vi "patientUpdateView.vi"() -> ()   [LabVIEW 2019]
doc: "40"
uses:
  03_Home/controller/logoutBtn.ctl
  03_Home/controller/exitBtn.ctl
  03_Home/controller/pannelState.ctl
  <vilib>/Utility/miscctls.llb/LVPointTypeDef.ctl
  subVI/patients_state.ctl
  globalValue.vi
panel:
  in  "patients_weight":dbl format="%.1f"
  in  "patients_age":dbl
  in  "patients_height":dbl format="%.1f"
  in  "patients_birthdate":dbl format="%<%Y-%m-%d>T"
  in  "cancelBtn":bool
  in  "patients_gender":string(combo)
  in  "backPage":bool
  in  "patients_info":string
  in  "patients_address":string
  in  "patients_phone":string
  in  "patients_email":string
  in  "patients_nm":string
  in  "updateBtn":bool
  in  "deleteBtn":bool
  out "patients_id":string
  out "userDetailInfo":string[](array[string])
  in  "Help Button":bool
  in  "LogOut Button":T1
  in  "Exit Button":T2
  out "userNm":string
  # "|"
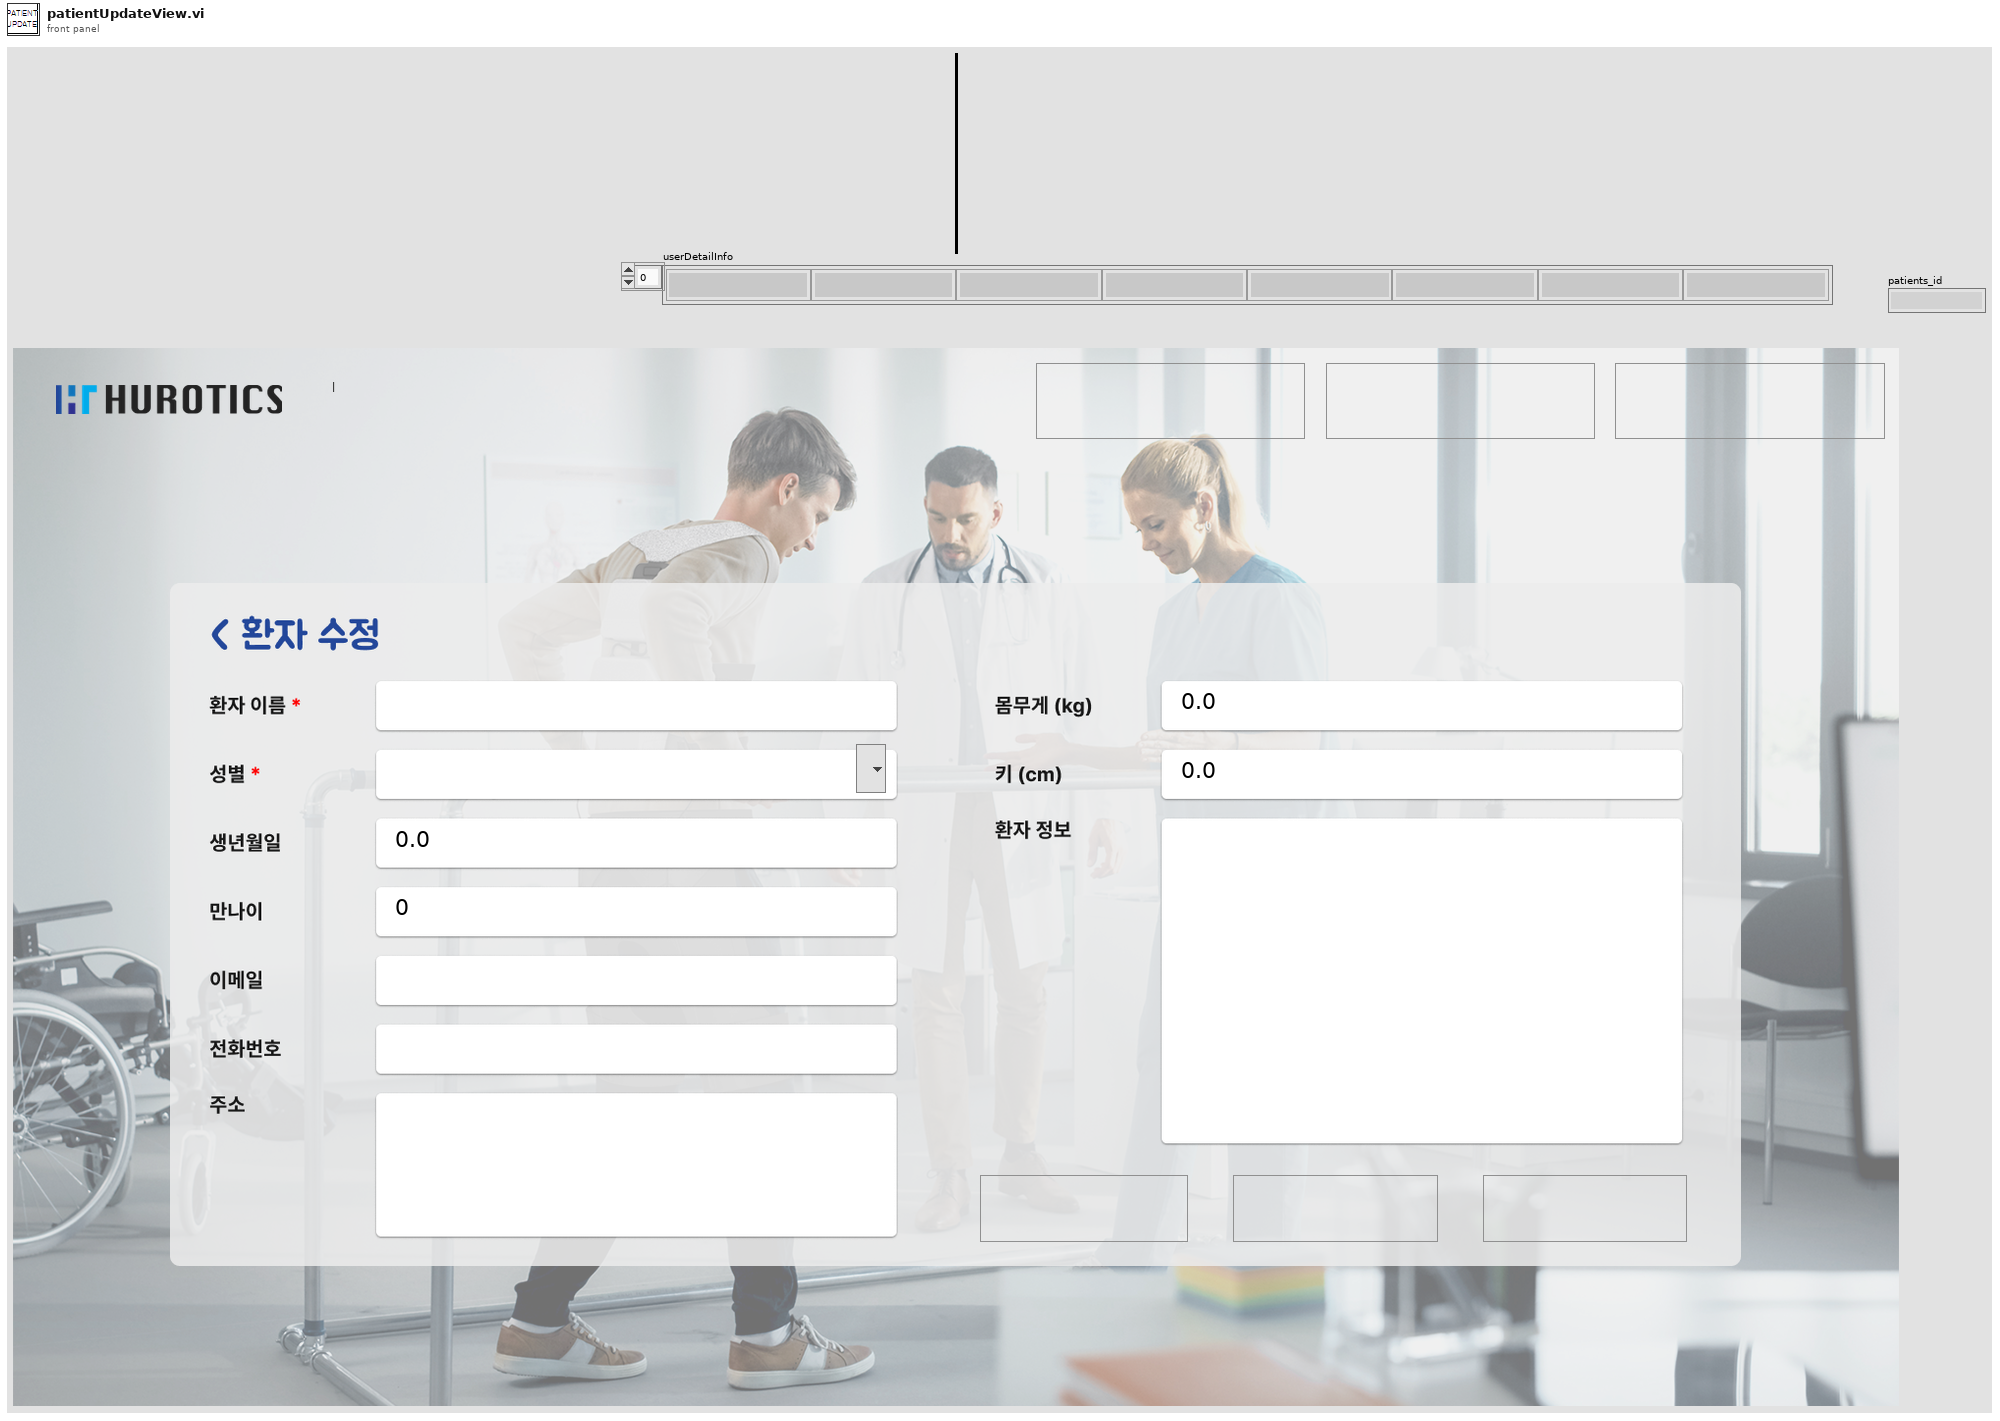
[diagram p1: front panel]
types:
  T1 = typedef "logoutBtn.ctl" = bool
  T2 = typedef "exitBtn.ctl" = bool
  T3 = typedef "pannelState.ctl" = enum16{"Init", "LogIn", "SignUpView", "Home", "Management_patientList", "Management_patientTrashtList", "Management_patientCreate", "Management_patientUpdate", "Management_patientTraining", "Management_patientTrainingDetail", "H-MEDI PatientList", "H-MEDI HardwareCtl", "Adjust", "FineTuning", "UserList", "UserDetail", "Exit"}
  T4 = typedef "LVPointTypeDef.ctl" = cluster{"Horizontal":i16, "Vertical":i16}
  T5 = enum16{"connection", "create", "getReadList", "getRead", "getCount", "update", "delete", "close"}
  T6 = typedef "patients_state.ctl" = enum16{"connection", "create", "getReadList", "getRead", "getCount", "update", "delete", "trash", "restore", "close"}
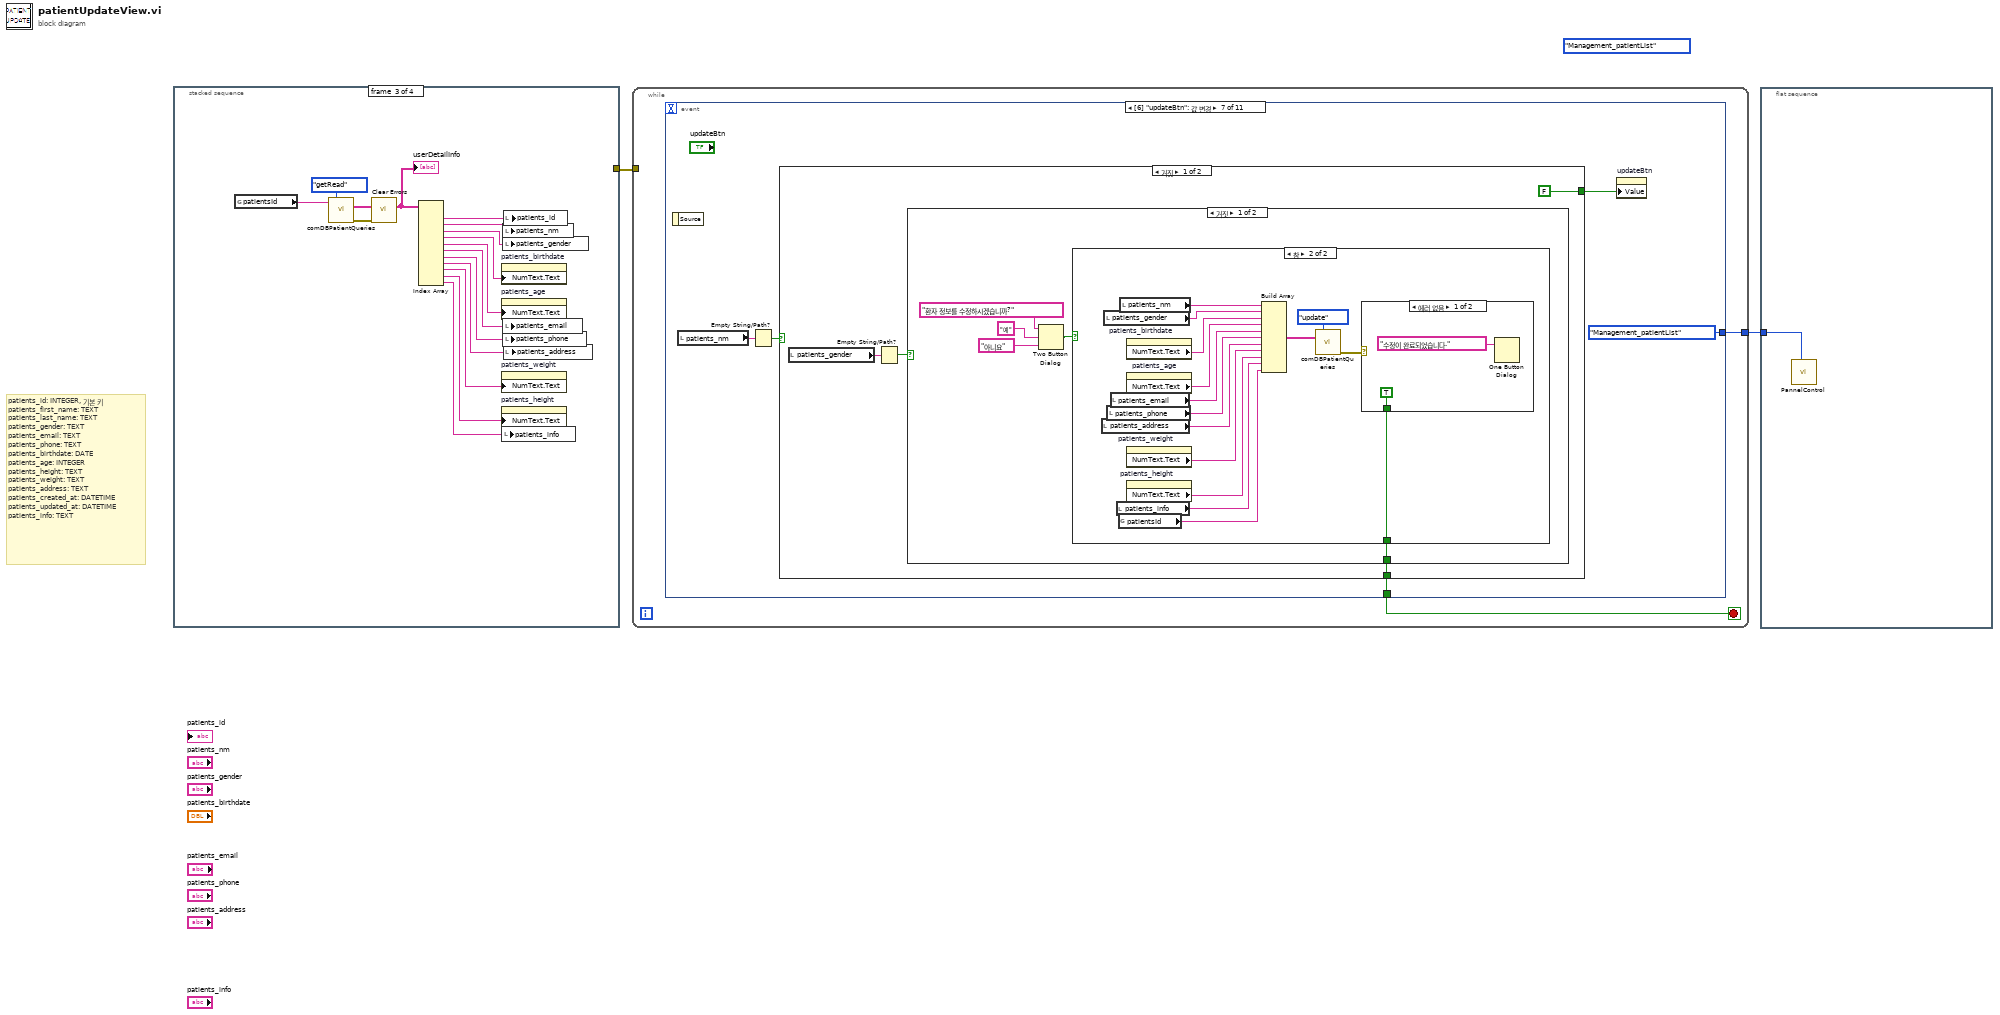
[diagram p0: block diagram]
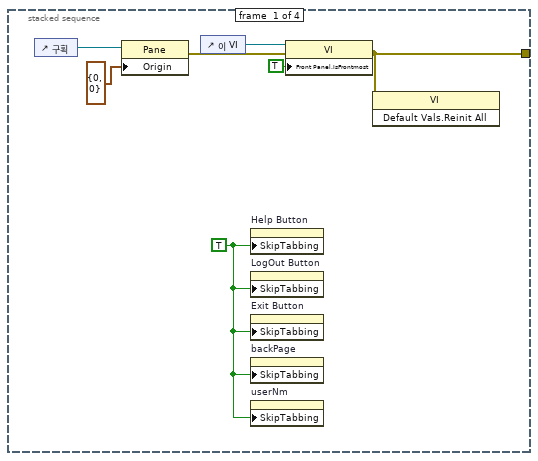
[diagram p2: hidden frame]
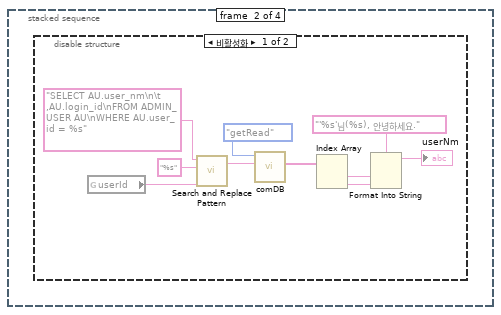
[diagram p3: hidden frame]
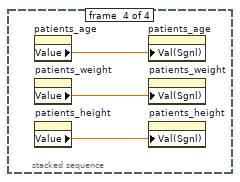
[diagram p5: hidden frame]
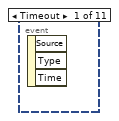
[diagram p6: hidden frame]
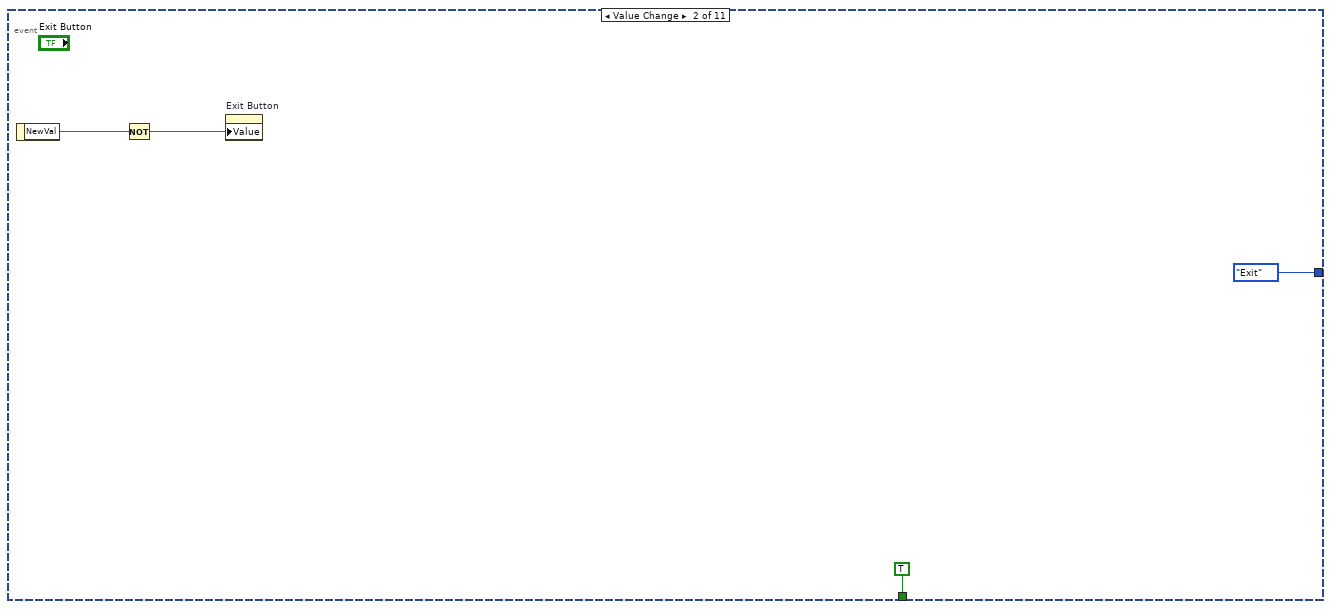
[diagram p7: hidden frame]
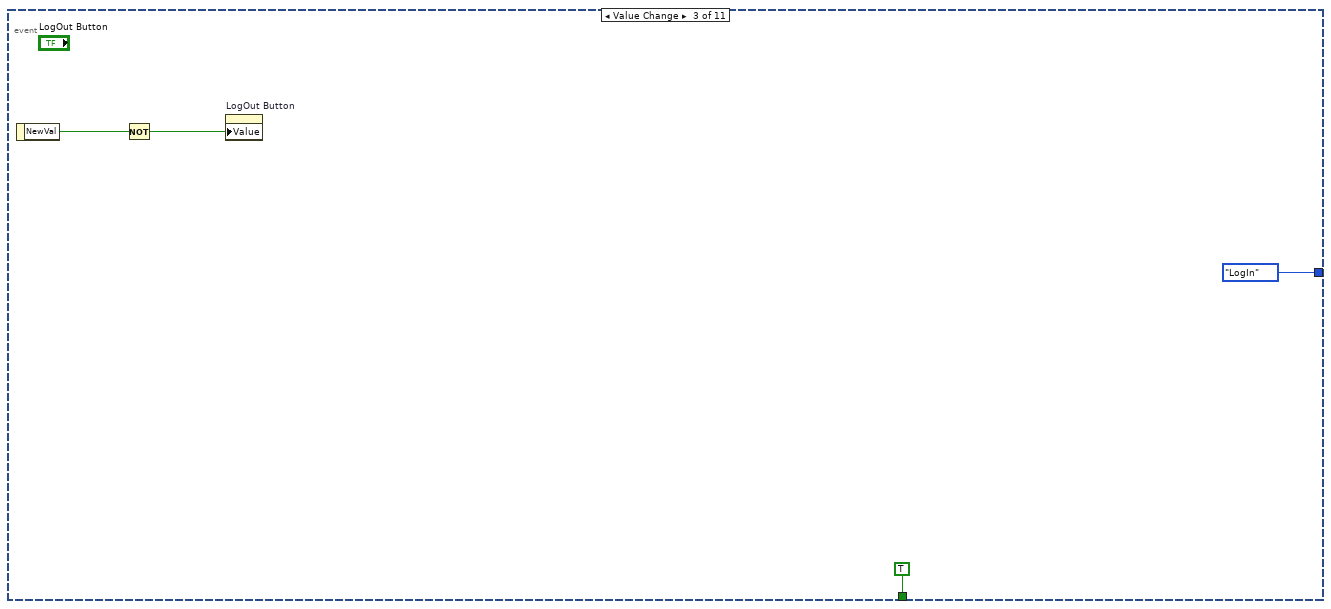
[diagram p8: hidden frame]
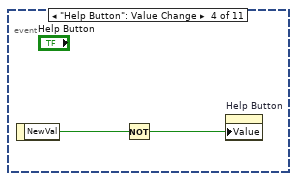
[diagram p9: hidden frame]
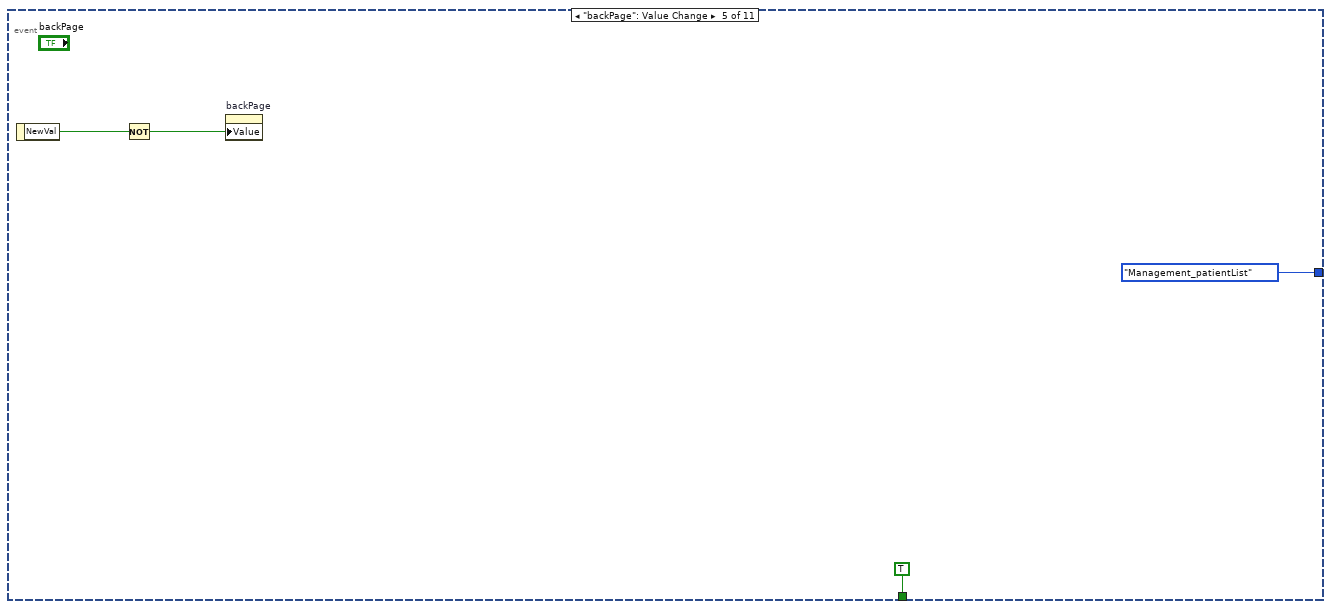
[diagram p10: hidden frame]
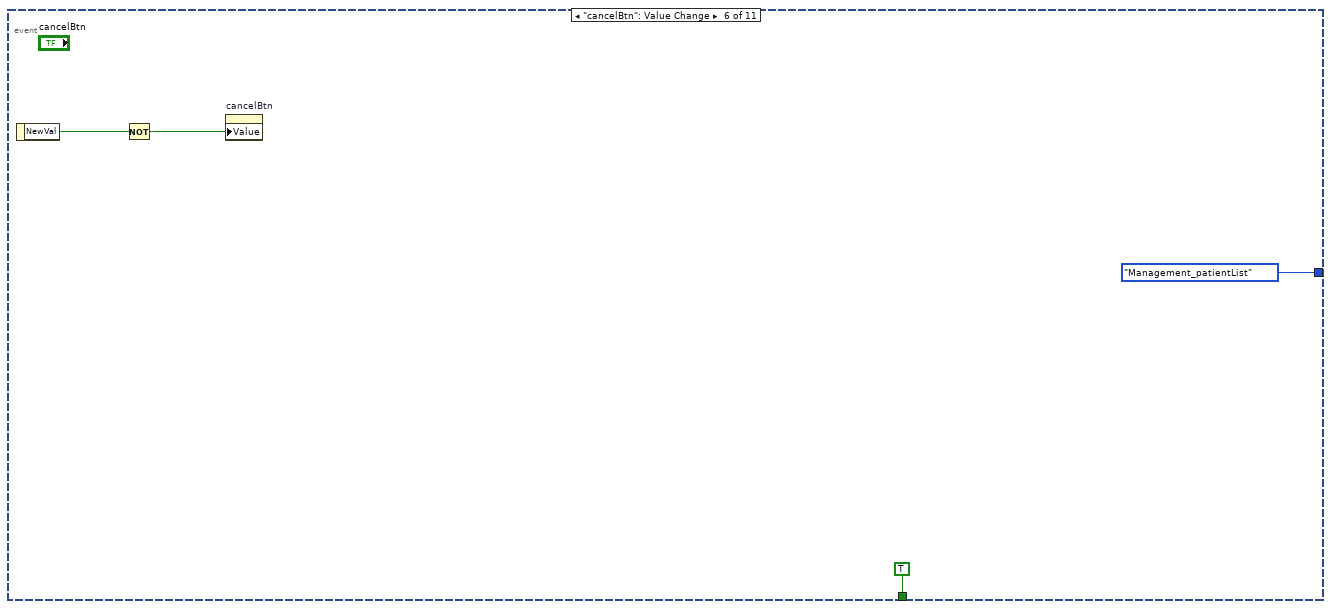
[diagram p11: hidden frame]
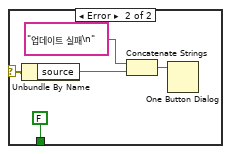
[diagram p13: hidden frame]
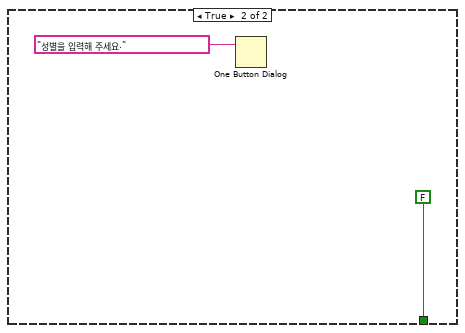
[diagram p14: hidden frame]
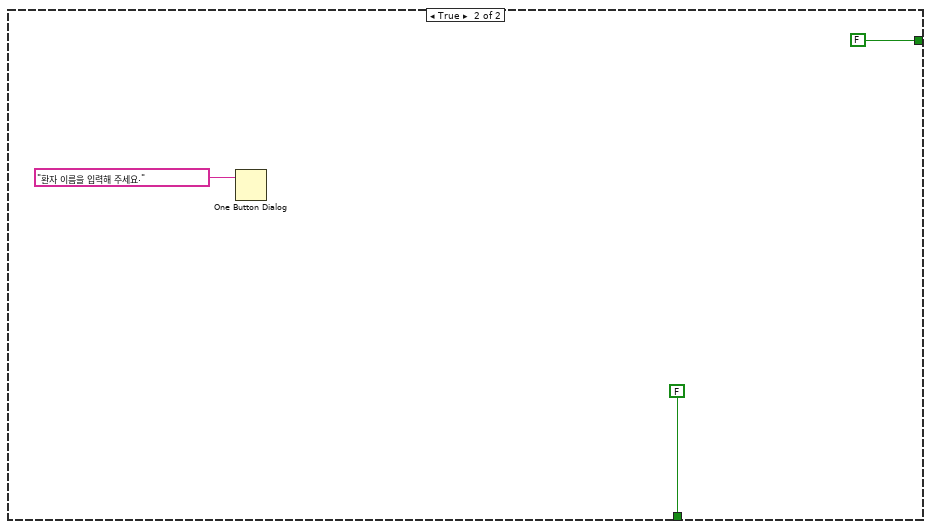
[diagram p15: hidden frame]
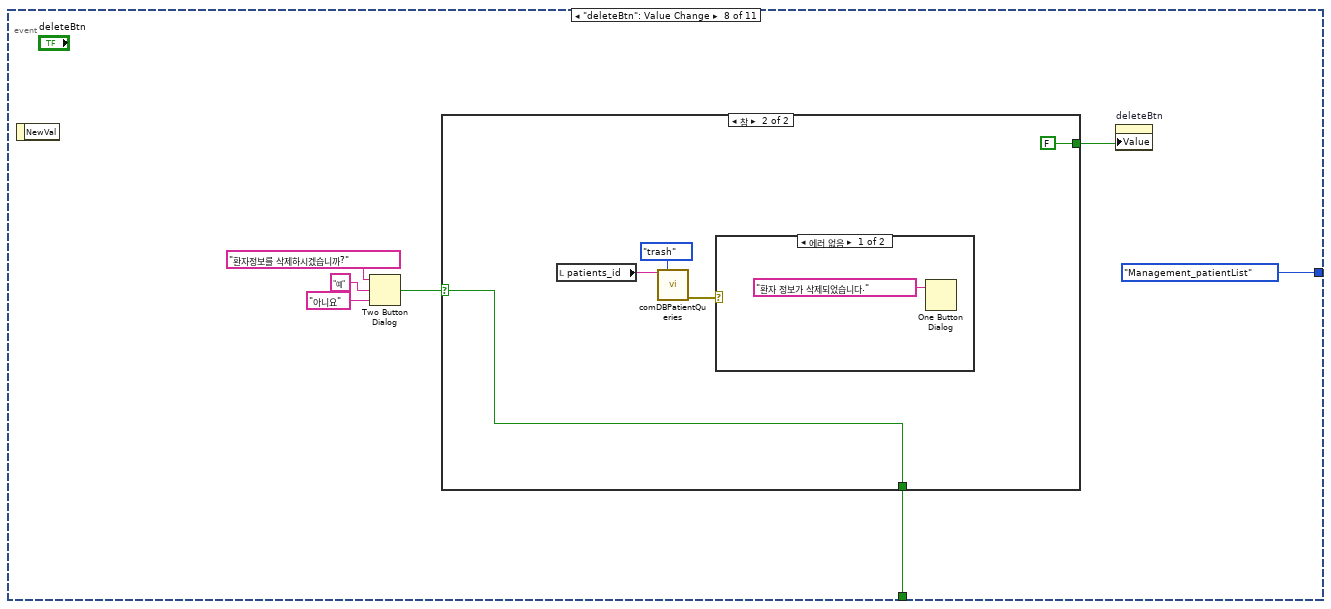
[diagram p16: hidden frame]
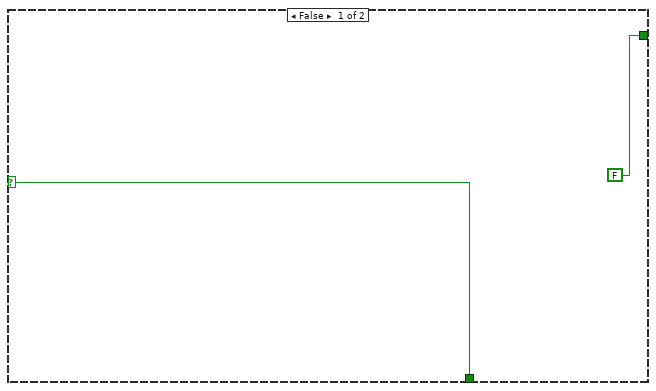
[diagram p17: hidden frame]
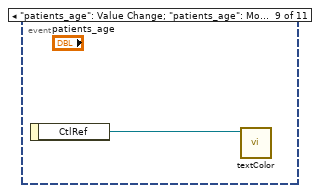
[diagram p19: hidden frame]
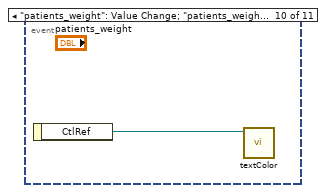
[diagram p20: hidden frame]
diagram:
  (unwired) pannelState."Management_patientList" ("State")
  # "patients_id: INTEGER, 기본 키\npatients_first_name: TEXT\npatients_last_name: TEXT\npatients_gender: TEXT\npatients_email: TEXT\npatients_phone: TEXT\npatients_birthdate: DATE\npatients_age: INTEGER\npatients_height: TEXT\npatients_weight: TEXT\npatients_address: TEXT\npatients_created_at: DATETIME\npatients_updated_at: DATETIME\npatients_info: TEXT"
  n1 = stacked-sequence {
    tunnel: [w4 _ _ _] -> w1
    frame #0 {
      w3 = TRUE ("탭으로 이동 시 건너뛰기")
      n2 = control-ref of="구획"() -> (w7:refnum<vi>)
      n3 = property class="Pane"(reference=w7, "Origin"=T4 {"Horizontal"=0, "Vertical"=0} ("원점")) -> (error out=w5:errorcluster)  [unwired: 1 in, 1 out]
      n4 = control-ref of="이 VI"() -> (w9:refnum<vi>)
      n5 = property on="Help Button" class="Bool (엄격한)"("SkipTabbing"=w3) -> ()  [unwired: 2 in, 2 out]
      n6 = property on="LogOut Button" class="Bool (엄격한)"("SkipTabbing"=w3) -> ()  [unwired: 2 in, 2 out]
      n7 = property on="Exit Button" class="Bool (엄격한)"("SkipTabbing"=w3) -> ()  [unwired: 2 in, 2 out]
      n8 = property on="backPage" class="Bool (엄격한)"("SkipTabbing"=w3) -> ()  [unwired: 2 in, 2 out]
      n9 = property on="userNm" class="Str"("SkipTabbing"=w3) -> ()  [unwired: 2 in, 2 out]
      n10 = property class="VI"(reference=w9, error in=w5, "Front Panel.IsFrontmost"=TRUE ("프런트패널 윈도우:맨 앞으로")) -> (error out=w4:errorcluster)  [unwired: 1 out]
      n11 = invoke class="VI" method="Default Vals.Reinit All"(error in=w4) -> ()  [unwired: 2 in, 3 out]
    }
    frame #1 {
      n12 = disable-structure shown="비활성화" {
        frame Disabled {
          n13 = global read "globalValue.vi" "userId"() -> (w10:string)
          n14 = call <vilib>:"Search and Replace Pattern.vi"("string"="SELECT AU.user_nm\n\t         ,AU.login_id\nFROM ADMIN_USER AU\nWHERE AU.user_id = %s" ("Query"), "regular expression (\"\")"="%s" ("regular expression (\"\")"), "replace string (\"\")"=w10) -> ("result string"=w11:string)  [unwired: 2 in, 1 out]
          n15 = call "comDB.vi"("Query"=w11, "State"=T5."getRead") -> ("result1DArray"=w17:string[])  [unwired: 5 in, 3 out]
          n16 = Index Array(array=w17) -> (element #1=w16:string, element #2=w15:string)  [unwired: 2 in]
          n17 = Format Into String(format string="'%s'님(%s), 안녕하세요." ("문자열"), w16, w15) -> (resulting string=→"userNm":string)  [unwired: 2 in, 1 out]
        }
        frame Enabled {
        }
      }
    }
    frame #2 {
      n18 = global read "globalValue.vi" "patientsId"() -> (w20:string)
      n19 = call "comDBPatientQueries.vi"("id"=w20, "State"=patients_state."getRead") -> ("result1DArray"=w28:string[], "error out"=w27:errorcluster)  [unwired: 10 in, 2 out]
      "userDetailInfo" <- w28
      n20 = call <vilib>:"Clear Errors.vi"("error in (no error)"=w27) -> ()  [unwired: 5 in, 2 out]
      n21 = Index Array(array=w28) -> (element #1=w29:string, element #2=w34:string, element #3=w26:string, element #4=w24:string, element #5=w23:string, element #6=w33:string, element #7=w32:string, element #8=w31:string, element #9=w22:string, element #10=w21:string, element #11=w30:string)  [unwired: 11 in]
      n22 = property on="patients_birthdate" class="DigNum (엄격한)"("NumText.Text"=w24) -> ()  [unwired: 2 in, 2 out]
      n23 = property on="patients_age" class="DigNum (엄격한)"("NumText.Text"=w23) -> ()  [unwired: 2 in, 2 out]
      n24 = property on="patients_weight" class="DigNum (엄격한)"("NumText.Text"=w22) -> ()  [unwired: 2 in, 2 out]
      n25 = property on="patients_height" class="DigNum (엄격한)"("NumText.Text"=w21) -> ()  [unwired: 2 in, 2 out]
      n26 = local write "patients_info"(w30) -> ()
      n27 = local write "patients_nm"(w34) -> ()
      n28 = local write "patients_gender"(w26) -> ()
      n29 = local write "patients_email"(w33) -> ()
      n30 = local write "patients_phone"(w32) -> ()
      n31 = local write "patients_id"(w29) -> ()
      n32 = local write "patients_address"(w31) -> ()
    }
    frame #3 {
      n33 = property on="patients_age" class="DigNum (엄격한)"() -> ("Value"=w37:dbl)  [unwired: 2 in, 2 out]
      n34 = property on="patients_weight" class="DigNum (엄격한)"() -> ("Value"=w36:dbl)  [unwired: 2 in, 2 out]
      n35 = property on="patients_height" class="DigNum (엄격한)"() -> ("Value"=w35:dbl)  [unwired: 2 in, 2 out]
      n36 = property on="patients_age" class="DigNum (엄격한)"("Val(Sgnl)"=w37) -> ()  [unwired: 2 in, 2 out]
      n37 = property on="patients_weight" class="DigNum (엄격한)"("Val(Sgnl)"=w36) -> ()  [unwired: 2 in, 2 out]
      n38 = property on="patients_height" class="DigNum (엄격한)"("Val(Sgnl)"=w35) -> ()  [unwired: 2 in, 2 out]
    }
  }
  n39 = while {
    tunnel: [w38] -> w2
    tunnel: w1 -> [_]
    stop <- w39 stop-if-true
    n40 = event shown="[6] \"updateBtn\": 값 변경" {
      selector: _ -> [_ _ _ _ _ _ _ _ _ _ _]
      dyn-events: _ -> [_ _ _ _ _ _ _ _ _ _ _]
      timeout: _ -> [_ _ _ _ _ _ _ _ _ _ _]
      tunnel: [_ TRUE TRUE _ TRUE TRUE w60 w101 _ _ _] -> w39
      tunnel: [_ pannelState."Exit" ("State") pannelState."LogIn" ("State") _ pannelState."Management_patientList" ("State") pannelState."Management_patientList" ("State") pannelState."Management_patientList" ("State") pannelState."Management_patientList" ("State") _ _ _] -> w38
      event Timeout {
        n41 = event-data() -> ()  [unwired: 1 in, 3 out]
      }
      event Value Change {
        n42 = event-data() -> ("NewVal"=w41:T2)  [unwired: 1 in]
        n43 = Not(x=w41) -> (.not. x?=w40:T2)
        n44 = property on="Exit Button" class="Bool (엄격한)"("Value"=w40) -> ()  [unwired: 2 in, 2 out]
      }
      event Value Change {
        n45 = event-data() -> ("NewVal"=w45:T1)  [unwired: 1 in]
        n46 = Not(x=w45) -> (.not. x?=w44:T1)
        n47 = property on="LogOut Button" class="Bool (엄격한)"("Value"=w44) -> ()  [unwired: 2 in, 2 out]
      }
      event "Help Button": Value Change {
        n48 = event-data() -> ("NewVal"=w49:bool)  [unwired: 1 in]
        n49 = Not(x=w49) -> (.not. x?=w48:bool)
        n50 = property on="Help Button" class="Bool (엄격한)"("Value"=w48) -> ()  [unwired: 2 in, 2 out]
      }
      event "backPage": Value Change {
        n51 = event-data() -> ("NewVal"=w52:bool)  [unwired: 1 in]
        n52 = Not(x=w52) -> (.not. x?=w51:bool)
        n53 = property on="backPage" class="Bool (엄격한)"("Value"=w51) -> ()  [unwired: 2 in, 2 out]
      }
      event "cancelBtn": Value Change {
        n54 = event-data() -> ("NewVal"=w57:bool)  [unwired: 1 in]
        n55 = Not(x=w57) -> (.not. x?=w55:bool)
        n56 = property on="cancelBtn" class="Bool (엄격한)"("Value"=w55) -> ()  [unwired: 2 in, 2 out]
      }
      event "updateBtn": Value Change {
        n57 = event-data() -> ()  [unwired: 1 in, 1 out]
        n58 = local read "patients_nm"() -> (w62:string)
        n59 = Empty String/Path?(string/path=w62) -> (empty?=w61:bool)
        n60 = case shown="거짓" w61 {
          tunnel: [FALSE ("createBtn") FALSE ("createBtn")] -> w59
          tunnel: [w63 FALSE] -> w60
          frame False {
            n61 = local read "patients_gender"() -> (w66:string)
            n62 = Empty String/Path?(string/path=w66) -> (empty?=w65:bool)
            n63 = case shown="거짓" w65 {
              tunnel: [w67 FALSE] -> w63
              frame False {
                n64 = Two Button Dialog(message="환자 정보를 수정하시겠습니까?" ("메시지"), 1:"아니요" ("거짓 버튼 이름(\"취소\")"), 2:"예" ("참 버튼 이름(\"확인\")")) -> (T button?=w68:bool)
                n65 = case shown="참" w68 {
                  selector: w68 -> [w72 _]
                  tunnel: [w72 w73] -> w67
                  frame False {
                  }
                  frame True {
                    n66 = local read "patients_address"() -> (w84:string)
                    n67 = local read "patients_gender"() -> (w81:string)
                    n68 = local read "patients_phone"() -> (w77:string)
                    n69 = local read "patients_email"() -> (w85:string)
                    n70 = local read "patients_info"() -> (w83:string)
                    n71 = global read "globalValue.vi" "patientsId"() -> (w74:string)
                    n72 = local read "patients_nm"() -> (w86:string)
                    n73 = property on="patients_birthdate" class="DigNum (엄격한)"() -> ("NumText.Text"=w79:string)  [unwired: 2 in, 2 out]
                    n74 = property on="patients_age" class="DigNum (엄격한)"() -> ("NumText.Text"=w78:string)  [unwired: 2 in, 2 out]
                    n75 = property on="patients_weight" class="DigNum (엄격한)"() -> ("NumText.Text"=w76:string)  [unwired: 2 in, 2 out]
                    n76 = property on="patients_height" class="DigNum (엄격한)"() -> ("NumText.Text"=w75:string)  [unwired: 2 in, 2 out]
                    n77 = Build Array(w86, w81, w79, w78, w85, w77, w84, w76, w75, w83, w74) -> (w82:string[])
                    n78 = call "comDBPatientQueries.vi"("State"=patients_state."update", "입력"=w82) -> ("error out"=w87:errorcluster)  [unwired: 10 in, 3 out]
                    n79 = case shown="에러 없음" w87 {
                      selector: w87 -> [_ w93]
                      tunnel: [TRUE FALSE] -> w73
                      frame No Error {
                        n80 = One Button Dialog(message="수정이 완료되었습니다." ("메시지")) -> ()  [unwired: 1 in, 1 out]
                      }
                      frame Error {
                        n81 = Unbundle By Name(w93) -> ("source"=w91:string)
                        n82 = Concatenate Strings("업데이트 실패\n", w91) -> (w92:string)
                        n83 = One Button Dialog(message=w92) -> ()  [unwired: 1 in, 1 out]
                      }
                    }
                  }
                }
              }
              frame True {
                n84 = One Button Dialog(message="성별을 입력해 주세요." ("메시지")) -> ()  [unwired: 1 in, 1 out]
              }
            }
          }
          frame True {
            n85 = One Button Dialog(message="환자 이름을 입력해 주세요." ("메시지")) -> ()  [unwired: 1 in, 1 out]
          }
        }
        n86 = property on="updateBtn" class="Bool (엄격한)"("Value"=w59) -> ()  [unwired: 2 in, 2 out]
      }
      event "deleteBtn": Value Change {
        n87 = event-data() -> ()  [unwired: 1 in, 1 out]
        n88 = Two Button Dialog(message="환자정보를 삭제하시겠습니까?" ("메시지"), 1:"아니요" ("거짓 버튼 이름(\"취소\")"), 2:"예" ("참 버튼 이름(\"확인\")")) -> (T button?=w103:bool)
        n89 = case shown="참" w103 {
          selector: w103 -> [w107 w109]
          tunnel: [FALSE ("deleteBtn") FALSE ("deleteBtn")] -> w102
          tunnel: [w107 w109] -> w101
          frame False {
          }
          frame True {
            n90 = local read "patients_id"() -> (w113:string)
            n91 = call "comDBPatientQueries.vi"("id"=w113, "State"=patients_state."trash") -> ("error out"=w112:errorcluster)  [unwired: 10 in, 3 out]
            n92 = case shown="에러 없음" w112 {
              frame No Error {
                n93 = One Button Dialog(message="환자 정보가 삭제되었습니다." ("메시지")) -> ()  [unwired: 1 in, 1 out]
              }
              frame Error {
              }
            }
          }
        }
        n94 = property on="deleteBtn" class="Bool (엄격한)"("Value"=w102) -> ()  [unwired: 2 in, 2 out]
      }
      event "patients_age": Value Change; "patients_age": Mouse Down {
        n95 = event-data() -> ("CtlRef"=w115:refnum<vi>)  [unwired: 1 in]
        n96 = call "textColor.vi"("디지털 입력"=w115) -> ()  [unwired: 11 in]
      }
      event "patients_weight": Value Change; "patients_weight": Mouse Down {
        n97 = event-data() -> ("CtlRef"=w116:refnum<vi>)  [unwired: 1 in]
        n98 = call "textColor.vi"("디지털 입력"=w116) -> ()  [unwired: 11 in]
      }
      event "patients_height": Value Change; "patients_height": Mouse Down {
        n99 = event-data() -> ("CtlRef"=w117:refnum<vi>)  [unwired: 1 in]
        n100 = call "textColor.vi"("디지털 입력"=w117) -> ()  [unwired: 11 in]
      }
    }
  }
  n101 = flat-sequence {
    tunnel: w2 -> [w118]
    frame #0 {
      n102 = call "PannelControl.vi"("State"=w118) -> ()  [unwired: 10 in, 1 out]
    }
  }
